vi "example setup for UIs - DO NOT RUN as is.vi"() -> ()   [LabVIEW 2020]
uses:
  <vilib>/Utility/miscctls.llb/LVRectTypeDef.ctl
  Basic FP Settings--cluster.ctl
panel:
  out "Original basic fp settings":T1
  out "Front Panel Window:Panel Bounds":T2
  # "DO NOT RUN THIS VI !"
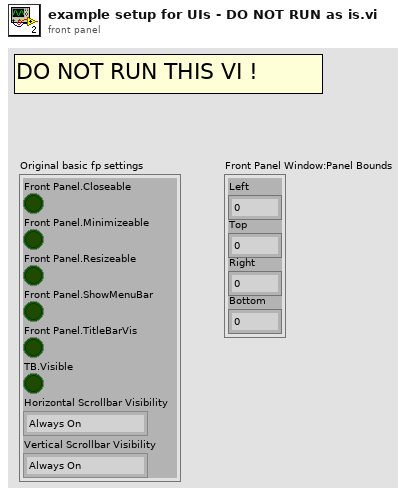
[diagram p1: front panel]
types:
  T1 = typedef "Basic FP Settings--cluster.ctl" = cluster{"Front Panel.Closeable":bool, "Front Panel.Minimizeable":bool, "Front Panel.Resizeable":bool, "Front Panel.ShowMenuBar":bool, "Front Panel.TitleBarVis":bool, "TB.Visible":bool, "Horizontal Scrollbar Visibility":enum16{"Always On", "Always Off", "Off While Running"}, "Vertical Scrollbar Visibility":enum16{"Always On", "Always Off", "Off While Running"}}
  T2 = typedef "LVRectTypeDef.ctl" = cluster{"Left":i16, "Top":i16, "Right":i16, "Bottom":i16}
  T3 = enum32{"Invalid", "Default", "Floating", "Floating/Auto-Hide", "Modal"}
  T4 = enum16{"Always On", "Always Off", "Off While Running"}
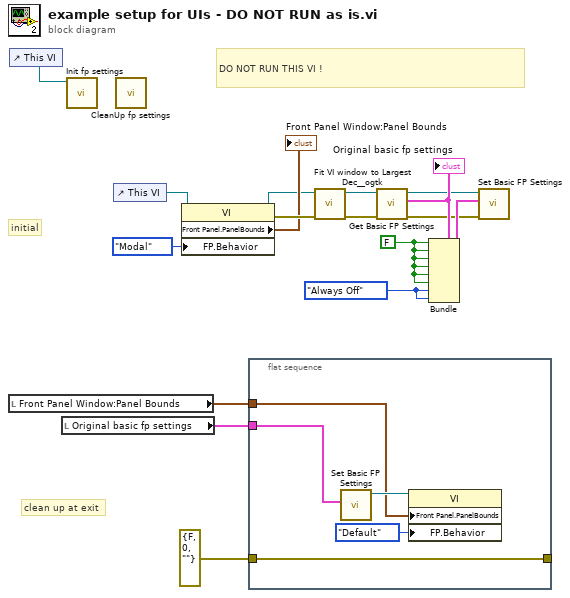
[diagram p0: block diagram]
diagram:
  w10 = T4."Always Off" ("Horizontal Scrollbar Visibility")
  w9 = FALSE ("Front Panel.Closeable")
  # "clean up at exit"
  # "initial"
  # "DO NOT RUN THIS VI !"
  n1 = local read "Front Panel Window:Panel Bounds"() -> (w3:T2)
  n2 = control-ref of="This VI"() -> (w1:refnum<vi>)
  n3 = local read "Original basic fp settings"() -> (w4:T1)
  n4 = call "Init fp settings.vi"("vi reference"=w1) -> ()  [unwired: 5 in, 4 out]
  n5 = control-ref of="This VI"() -> (w13:refnum<vi>)
  n6 = call "CleanUp fp settings.vi"() -> ()  [unwired: 8 in, 2 out]
  n7 = property class="VI"(reference=w13, "FP.Behavior"=T3."Modal" ("Front Panel Window:Behavior")) -> (reference out=w14:refnum<vi>, error out=w16:errorcluster, "Front Panel.PanelBounds"=→"Front Panel Window:Panel Bounds":T2)  [unwired: 1 in]
  n8 = flat-sequence {
    tunnel: w4 -> [w20]
    tunnel: w3 -> [w19]
    tunnel: [w18] -> _
    tunnel: errorcluster {"status"=FALSE, "code"=0, "source"=""} ("error out") -> [w18]
    frame #0 {
      n9 = call "Set Basic FP Settings.vi"("basic fp settings"=w20) -> ("vi reference out"=w22:refnum<vi>)  [unwired: 9 in, 1 out]
      n10 = property class="VI"(reference=w22, "Front Panel.PanelBounds"=w19, "FP.Behavior"=T3."Default" ("Front Panel Window:Behavior")) -> ()  [unwired: 1 in, 2 out]
    }
  }
  n11 = call <userlib>:"Fit VI window to Largest Dec__ogtk.vi"("error in (no error)"=w16, "VI Ref (calling VI)"=w14) -> ("error out"=w5:errorcluster, "dup VI Ref"=w17:refnum<vi>)  [unwired: 4 in]
  n12 = call "Get Basic FP Settings.vi"("error in (no error)"=w5, "vi reference"=w17) -> ("error out"=w6:errorcluster, "basic fp settings"=w8:T1, "vi reference out"=w7:refnum<vi>)  [unwired: 7 in]
  "Original basic fp settings" <- w8
  n13 = Bundle(cluster=w8, "Front Panel.Closeable"=w9, "Front Panel.Minimizeable"=w9, "Front Panel.Resizeable"=w9, "Front Panel.ShowMenuBar"=w9, "Front Panel.TitleBarVis"=w9, "TB.Visible"=w9, "Horizontal Scrollbar Visibility"=w10, "Vertical Scrollbar Visibility"=w10) -> (w11:T1)
  n14 = call "Set Basic FP Settings.vi"("error in (no error)"=w6, "basic fp settings"=w11, "vi reference"=w7) -> ()  [unwired: 7 in, 2 out]
